vi "小三轮的 RT Main.vi"() -> ()   [LabVIEW 2017]
doc: "The myRIO Custom FPGA Project template acquires button data from the onboard button and displays the button value on a Boolean indicator. The SYS.RDY indicator shows the FPGA status."
uses:
  <vilib>/Platform/TimedLoop/XDataNode/timing_clust.ctl
  <vilib>/Platform/TimedLoop/XDataNode/nitl_modes.ctl
  <vilib>/Platform/TimedLoop/XDataNode/wakeup.ctl
  <vilib>/myRIO/Instrument Drivers/Onboard IO/PWM/vis/Set Duty Cycle and Frequency.vi
  <vilib>/myRIO/Common/Instrument Driver Framework/myRIO v1.0/UART/vis/myRIO v1.0 Close UART.vi
  <vilib>/Utility/error.llb/Error Cluster From Error Code.vi
  <vilib>/rvi/errors/niLvFpgaAdjustHostInterfaceError.vi
  <vilib>/myRIO/Common/Instrument Driver Framework/myRIO v1.0/Encoder/vis/myRIO v1.0 Read Encoder.vi
  <vilib>/myRIO/Common/Instrument Driver Framework/myRIO v1.0/PWM/vis/myRIO v1.0 Write PWM.vi
  <vilib>/myRIO/Common/Instrument Driver Framework/myRIO v1.0/DIO/vis/myRIO v1.0 Write DIO.vi
  <vilib>/FPGAPlugInAG/Dynamic/niLvFpga_Close_Dynamic.vi
  <vilib>/myRIO/Common/Instrument Driver Framework/Utilities/vis/FPGA Ref Manager.vi
  <vilib>/myRIO/Common/Instrument Driver Framework/myRIO v1.0/myRIO v1.0 Reset FPGA.vi
  <vilib>/myRIO/Common/Instrument Driver Framework/myRIO v1.0/IRQ/vis/myRIO v1.0 IRQ Info FGV.vi
  <vilib>/myRIO/Common/Instrument Driver Framework/myRIO v1.0/IRQ/vis/myRIO v1.0 Timer IRQ Info FGV.vi
  <vilib>/myRIO/Common/Instrument Driver Framework/myRIO v1.0/IRQ/vis/myRIO v1.0 ISR Agent.vi
  <vilib>/Platform/TimedLoop/XDataNode/XDataNode.xnode
  <vilib>/rvi/interface/nirviReadWriteControl/nirviReadWriteControl.xnode
  <vilib>/rvi/interface/nirviCloseFPGA/nirviCloseFPGA.xnode
  <vilib>/Platform/TimedLoop/XDataNode/XDNodeRunTimeDep.lvlib
  <vilib>/myRIO/Instrument Drivers/Onboard IO/PWM/PWM.lvlib
  <vilib>/myRIO/Instrument Drivers/Onboard IO/DIO/DIO.lvlib
  <vilib>/myRIO/Instrument Drivers/Onboard IO/Encoder/Encoder.lvlib
  <vilib>/myRIO/Instrument Drivers/Utilities/Utilities.lvlib
  NiFpgaLv.dll
  <vilib>/rvi/interface/Simulation/niFpgaSimulationCallBeginRW.vi
panel:
  out "error out":errorcluster
  out "pulse width (uSec) 2":u32
  out "pulse width (uSec)":u32
  out "ENC2":i32
  out "ENC1":i32
  in  "停止":bool
  out "ENC":i32[](array[numeric])
  in  "DIR":bool[](array[boolean])=[TRUE, TRUE, TRUE, TRUE, FALSE, FALSE]
  in  "PWM":dbl[](array[numeric])=[1.0, 1.0, 1.0, 1.0]
  in  "舵机":dbl[](array[numeric])=[0.0, 0.0, 0.0]
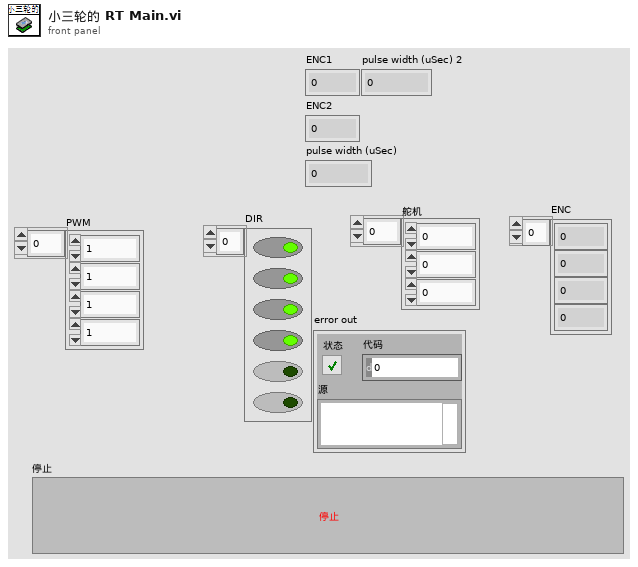
[diagram p1: front panel]
types:
  T1 = typedef "XDNodeRunTimeDep.lvlib/timing_clust.ctl" = cluster{"Expected End [f-1]":u64, "Actual End [f-1]":u64, "Finished Late? [f-1]":bool, "Expected End [i-1]":u64, "Actual End [i-1]":u64, "Finished Late? [i-1]":bool, "Expected Start [i]":u64, "Actual Start [i]":u64, "Expected Start [f]":u64, "Actual Start [f]":u64, "Source Name":string, "Structure Name":string, "Period":i64, "Deadline":i64, "Offset":i64, "Start":i64, "Priority":i32, "Timeout":i32, "Mode":T2, "Wakeup Reason":T3, "Error":errorcluster, "Source Type":string, "Secondary Source Type":string, "Global End Time":u64, "Global Start Time":u64, "Frame Duration":u64, "Iteration Duration":u64, "Assigned CPU":i32, "I/O Scan Engine Mode":u32}
  T2 = typedef "XDNodeRunTimeDep.lvlib/nitl_modes.ctl" = enum32{"No Change", "Process missed periods, maintain original phase", "Discard missed periods, maintain original phase", "Process missed periods, ignore original phase", "Discard missed periods, ignore original phase"}
  T3 = typedef "XDNodeRunTimeDep.lvlib/wakeup.ctl" = enum32{"Normal", "Aborted", "Asynchronous wakeup", "Timing source error", "Timed loop error", "Timeout"}
  T4 = typedef "PWM.lvlib/PWM Reference.ctl" = cluster{"myRIO Reference":T5, "PWM Channels Enum":T9, "PWM Configuration":T10}
  T5 = typedef "myRIO Generic Hardware Reference.ctl" = cluster{"myRIO Model":T6, "myRIO Hardware Reference":T7}
  T6 = typedef "Hardware Version Enum.ctl" = enum16{"Unknown", "myRIO-1900", "myRIO-1950", "roboRIO", "NI ELVIS RIO CM"}
  T7 = typedef "myRIO v1.0 Reference.ctl" = cluster{"Generic FPGA Reference":T8, "Allow multiple opens":bool}
  T8 = typedef "Generic FPGA Reference.ctl" = refnum<k20>
  T9 = typedef "PWM Channels Enum.ctl" = enum16{"Not Connected", "C/PWM0", "C/PWM1", "A/PWM0", "A/PWM1", "A/PWM2", "B/PWM0", "B/PWM1", "B/PWM2", "PWM/PWM0", "PWM/PWM1", "PWM/PWM2", "PWM/PWM3", "PWM/PWM4", "PWM/PWM5", "PWM/PWM6", "PWM/PWM7", "PWM/PWM8", "PWM/PWM9"}
  T10 = typedef "PWM.lvlib/PWM Configuration.ctl" = cluster{"Frequency":dbl, "Duty Cycle":dbl}
  T11 = typedef "Encoder.lvlib/Encoder Reference.ctl" = cluster{"myRIO Reference":T5, "Encoder Channels Enum":T12}
  T12 = typedef "Encoder Channels Enum.ctl" = enum16{"Not Connected", "C/ENC0", "C/ENC1", "A/ENC", "B/ENC", "DIO/ENC0", "DIO/ENC1", "DIO/ENC2", "DIO/ENC3", "DIO/ENC4"}
  T13 = typedef "DIO.lvlib/DIO Reference.ctl" = cluster{"myRIO Reference":T5, "DIO Channels List":T14}
  T14 = typedef "DIO Channels List.ctl" = T15[]
  T15 = typedef "DIO Channels Enum.ctl" = enum16{"Not Connected", "C/DIO0", "C/DIO1", "C/DIO2", "C/DIO3", "C/DIO4", "C/DIO5", "C/DIO6", "C/DIO7", "A/DIO0", "A/DIO1", "A/DIO2", "A/DIO3", "A/DIO4", "A/DIO5", "A/DIO6", "A/DIO7", "A/DIO8", "A/DIO9", "A/DIO10", "A/DIO11", "A/DIO12", "A/DIO13", "A/DIO14", "A/DIO15", "B/DIO0", "B/DIO1", "B/DIO2", "B/DIO3", "B/DIO4", "B/DIO5", "B/DIO6", "B/DIO7", "B/DIO8", "B/DIO9", "B/DIO10", "B/DIO11", "B/DIO12", "B/DIO13", "B/DIO14", "B/DIO15", "LED0", "LED1", "LED2", "LED3", "Button0", "DIO/DIO0", "DIO/DIO1", "DIO/DIO2", "DIO/DIO3", "DIO/DIO4", "DIO/DIO5", "DIO/DIO6", "DIO/DIO7", "DIO/DIO8", "DIO/DIO9", "SPI/CS0", "SPI/CS1", "SPI/CS2", "SPI/CS3", "LED RADIO (Green)", "LED RADIO (Red)", "LED COMM (Green)", "LED COMM (Red)", "LED MODE (Green)", "LED MODE (Red)"}
  T16 = cluster{"舵机":T4[], "PWM":T4[], "ENC":T11[], "DIR":T13, "error out":errorcluster, "FPGA VI引用输出":refnum<k20>}
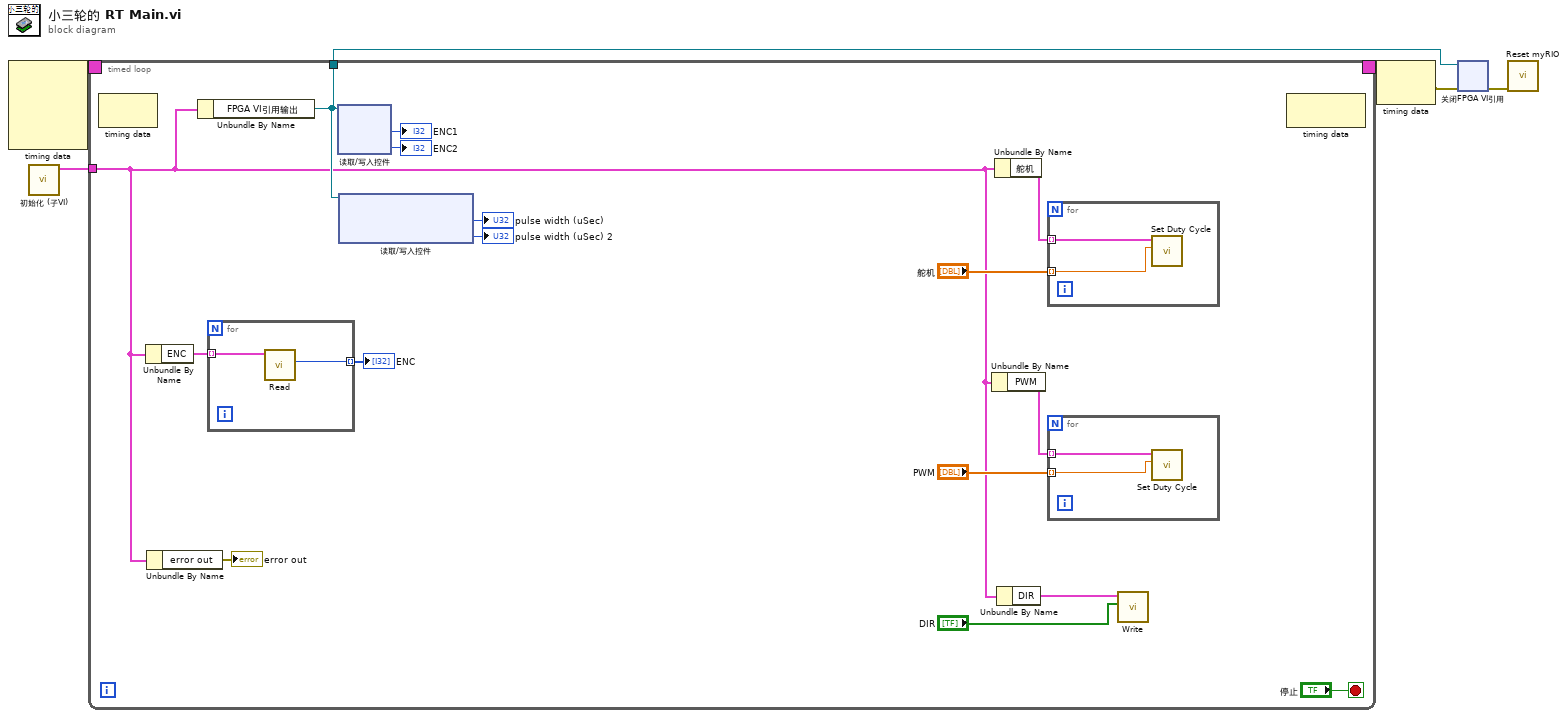
[diagram p0: block diagram]
diagram:
  n1 = node-c288() -> (w6:T1)  [unwired: 4 in]
  n2 = call "初始化 (子VI).vi"() -> ("输出簇"=w4:T16)  [unwired: 11 in]
  n3 = timed-loop {
    timing: w6 -> [_]
    timing-out: [_] -> w5
    tunnel: w4 -> [w8]
    tunnel: [w11] -> w1
    stop <- "停止" stop-if-true
    n4 = node-c288() -> ()  [unwired: 1 in, 1 out]
    n5 = Unbundle By Name(w8) -> ("ENC"=w19:T11[])
    n6 = Unbundle By Name(w8) -> ("error out"=→"error out":errorcluster)
    n7 = Unbundle By Name(w8) -> ("FPGA VI引用输出"=w11:refnum<k20>)
    n8 = for {
      tunnel: w19 -> [w24] mode=indexing
      tunnel: [w23] -> w15 mode=indexing
      n9 = call <vilib>:"Read.vi"("Encoder Ref In"=w24) -> ("Counter Value"=w23:i32)  [unwired: 6 in, 4 out]
    }
    "ENC" <- w15
    n10 = xnode "读取/写入控件"("FPGA VI引用输入"=w11) -> ("ENC1"=→"ENC1":i32, "ENC2"=→"ENC2":i32)  [unwired: 1 in, 2 out]
    n11 = xnode "读取/写入控件"("FPGA VI引用输入"=w11) -> ("pulse width (uSec)"=→"pulse width (uSec)":u32, "pulse width (uSec) 2"=→"pulse width (uSec) 2":u32)  [unwired: 1 in, 2 out]
    n12 = Unbundle By Name(w8) -> ("PWM"=w22:T4[])
    n13 = Unbundle By Name(w8) -> ("舵机"=w20:T4[])
    n14 = Unbundle By Name(w8) -> ("DIR"=w21:T13)
    n15 = for {
      tunnel: w20 -> [w26] mode=indexing
      tunnel: "舵机" -> [w25] mode=indexing
      n16 = call <vilib>:"Set Duty Cycle.vi"("Duty Cycle"=w25, "PWM Ref In"=w26) -> ()  [unwired: 7 in, 2 out]
    }
    n17 = for {
      tunnel: w22 -> [w28] mode=indexing
      tunnel: "PWM" -> [w27] mode=indexing
      n18 = call <vilib>:"Set Duty Cycle.vi"("Duty Cycle"=w27, "PWM Ref In"=w28) -> ()  [unwired: 7 in, 2 out]
    }
    n19 = call <vilib>:"Write.vi"("Values"="DIR", "DIO Ref In"=w21) -> ()  [unwired: 7 in, 2 out]
    n20 = node-c288() -> ()  [unwired: 1 in, 1 out]
  }
  n21 = node-c288(w5) -> (w3:errorcluster)
  n22 = xnode "关闭FPGA VI引用"("FPGA VI引用输入"=w1, "错误输入"=w3) -> ("错误输出"=w2:errorcluster)
  n23 = call <vilib>:"Reset myRIO.vi"("error in (no error)"=w2) -> ()  [unwired: 10 in, 1 out]
